vi "run_chatcompletion_wrap.vi"(8 "error in (no error)":errorcluster, 10 "Messages":refnum<class "abstract_message_base.lvclass">[](array[class]), 11 "abstract_llm_chatcompletion in":refnum<class "abstract_llm_base.lvclass">) -> (0 "error out":errorcluster, 2 "Response":refnum<class "abstract_message_base.lvclass">, 3 "abstract_llm_chatcompletion out":refnum<class "abstract_llm_base.lvclass">)   [LabVIEW 2020, in "abstract_llm_chatcompletion.lvclass"]
uses:
  abstract_llm_chatcompletion.lvclass
  abstract_llm_base/abstract_llm_base.lvclass
  abstract_message_base/abstract_message_base.lvclass
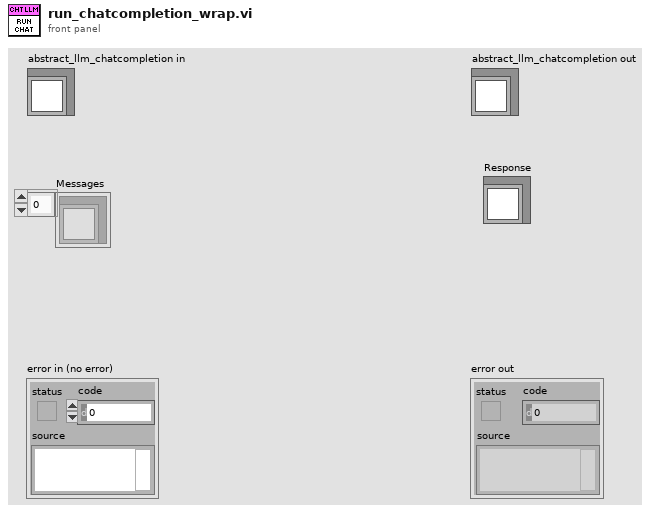
[diagram p1: front panel]
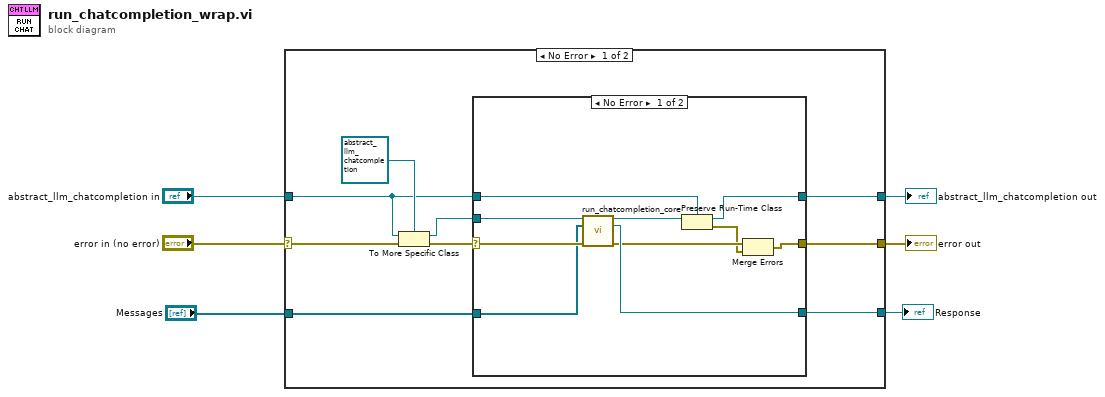
[diagram p0: block diagram]
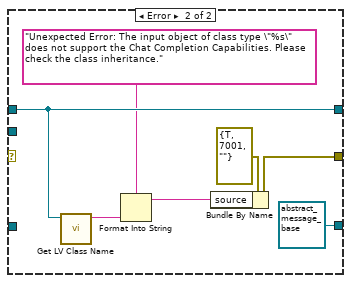
[diagram p2: hidden frame]
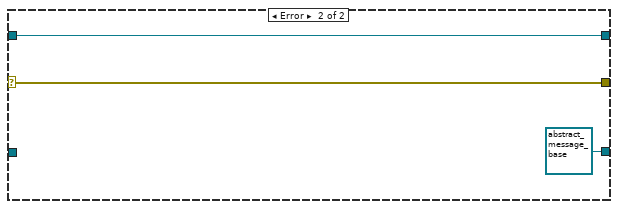
[diagram p3: hidden frame]
diagram:
  n1 = case shown="No Error" "error in (no error)" {
    selector: "error in (no error)" -> [w10 w35]
    tunnel: [w7 w35] -> w5
    tunnel: [w8 w34] -> w3
    tunnel: "abstract_llm_chatcompletion in" -> [w9 w34]
    tunnel: "Messages" -> [w12 _]
    tunnel: [w11 refnum<class "abstract_message_base.lvclass"> refnum ("Response")] -> w1
    frame No Error {
      n2 = To More Specific Class(target class=refnum<class "abstract_llm_chatcompletion.lvclass"> refnum ("abstract_llm_chatcompletion.lvclass"), reference=w9, error in=w10) -> (specific class reference=w13:refnum<class "abstract_llm_chatcompletion.lvclass">, error out=w14:errorcluster)
      n3 = case shown="No Error" w14 {
        selector: w14 -> [w25 _]
        tunnel: w13 -> [w24 _]
        tunnel: w12 -> [w23 _]
        tunnel: [w22 refnum<class "abstract_message_base.lvclass"> refnum ("Response")] -> w11
        tunnel: w9 -> [w20 w31]
        tunnel: [w19 w31] -> w8
        tunnel: [w16 w29] -> w7
        frame No Error {
          n4 = call-dynamic "run_chatcompletion_core.vi"("chatcompletion_llm_interface in"=w24, "Messages"=w23, "error in (no error)"=w25) -> ("chatcompletion_llm_interface out"=w21:refnum<class "abstract_llm_chatcompletion.lvclass">, "Response"=w22:refnum<class "abstract_message_base.lvclass">, "error out"=w18:errorcluster)  [unwired: 10 in]
          n5 = Preserve Run-Time Class(object in=w21, 2:w20) -> (object out=w19:refnum<class "abstract_llm_base.lvclass">, error out=w17:errorcluster)  [unwired: 1 in]
          n6 = Merge Errors(w18, w17) -> (w16:errorcluster)
        }
        frame Error {
          n7 = call <vilib>:"Get LV Class Name.vi"("object"=w31) -> ("class name"=w27:string)  [unwired: 9 in, 1 out]
          n8 = Format Into String(format string="Unexpected Error: The input object of class type \"%s\" does not support the Chat Completion Capabilities. Please check the class inheritance.", w27) -> (resulting string=w26:string)  [unwired: 2 in, 1 out]
          n9 = Bundle By Name(cluster=errorcluster {"status"=TRUE, "code"=7001, "source"=""} ("error constant"), "source"=w26) -> (w29:errorcluster)
        }
      }
    }
    frame Error {
    }
  }
  "error out" <- w5
  "abstract_llm_chatcompletion out" <- w3
  "Response" <- w1
